vi "Get Recording.vi"(8 "error in":errorcluster, 9 "Get":bool, 10 "Recording":fxp<+/-,8,8>[](array[numeric]), 11 "Interface In":T1) -> (0 "error out":errorcluster, 1 "Get?":bool, 3 "Interface Out":T1)   [LabVIEW 2015]
uses:
  TypeDefs Host/FPGA Dynamic Interface.ctl
  TypeDefs Host/Open Audio FGV Enum.ctl
  <vilib>/Utility/error.llb/Error Cluster From Error Code.vi
  <vilib>/rvi/errors/niLvFpgaAdjustHostInterfaceError.vi
  <vilib>/rvi/interface/common/niFpgaWaitOnOcc.vi
  <vilib>/rvi/interface/nirviReadWriteControl/nirviReadWriteControl.xnode
  <vilib>/rvi/interface/nirviMethod/nirviMethod.xnode
  <vilib>/rvi/errors/niLvFpgaMergeErrorWithErrorCode.vi
  <vilib>/FPGAPlugInAG/Dynamic/niLvFpga_WriteFifo_Dynamic.vi
  NiFpgaLv.dll
  <vilib>/rvi/interface/Simulation/niFpgaSimulationCallBeginRW.vi
  <vilib>/FPGAPlugInAG/Dynamic/niLvFpga_ConfigureFifo_Dynamic.vi
  <vilib>/FPGAPlugInAG/Dynamic/niLvFpga_StartFifo_Dynamic.vi
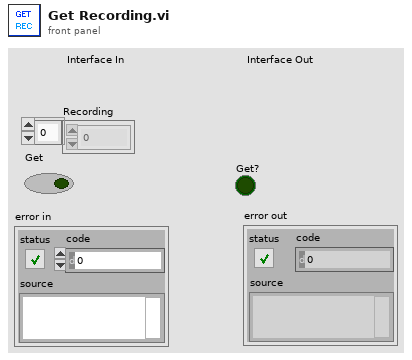
[diagram p1: front panel]
types:
  T1 = typedef "FPGA Dynamic Interface.ctl" = refnum<k20>
  T2 = typedef "Open Audio FGV Enum.ctl" = enum16{"Get", "Set"}
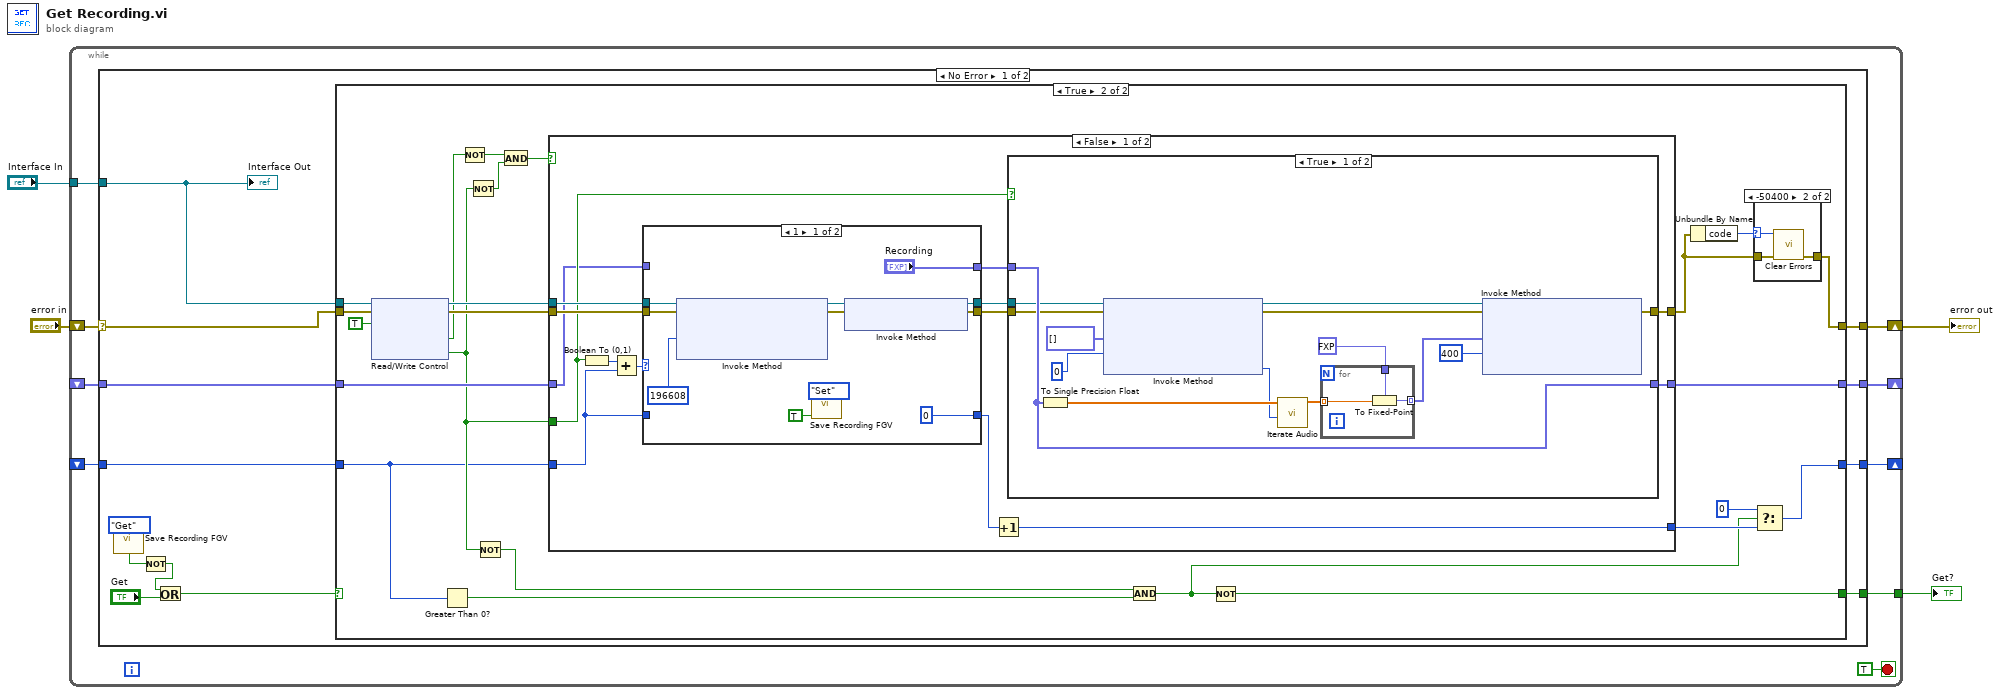
[diagram p0: block diagram]
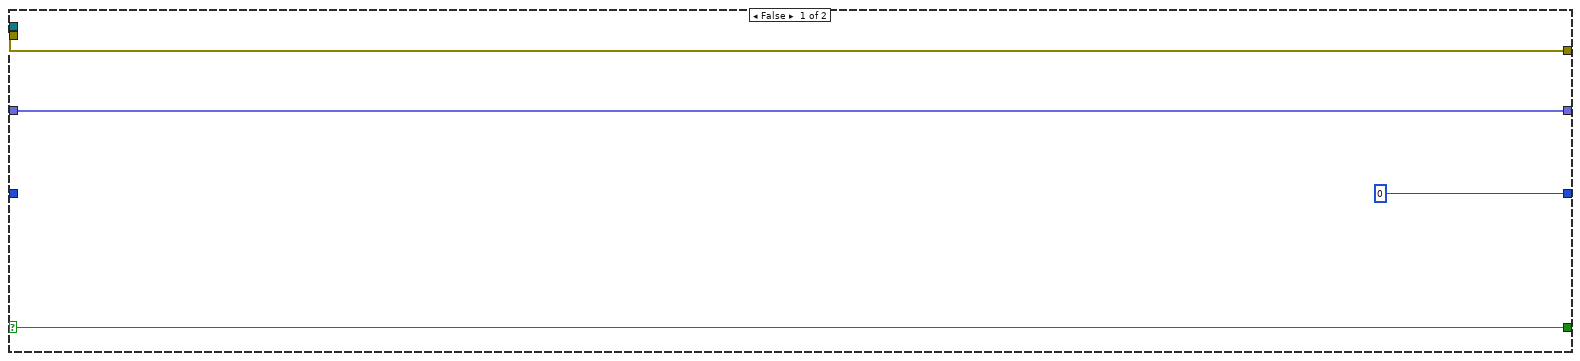
[diagram p2: hidden frame]
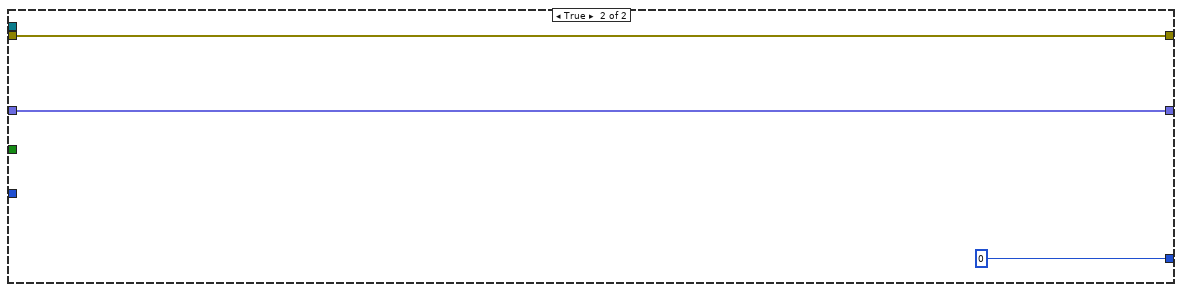
[diagram p6: hidden frame]
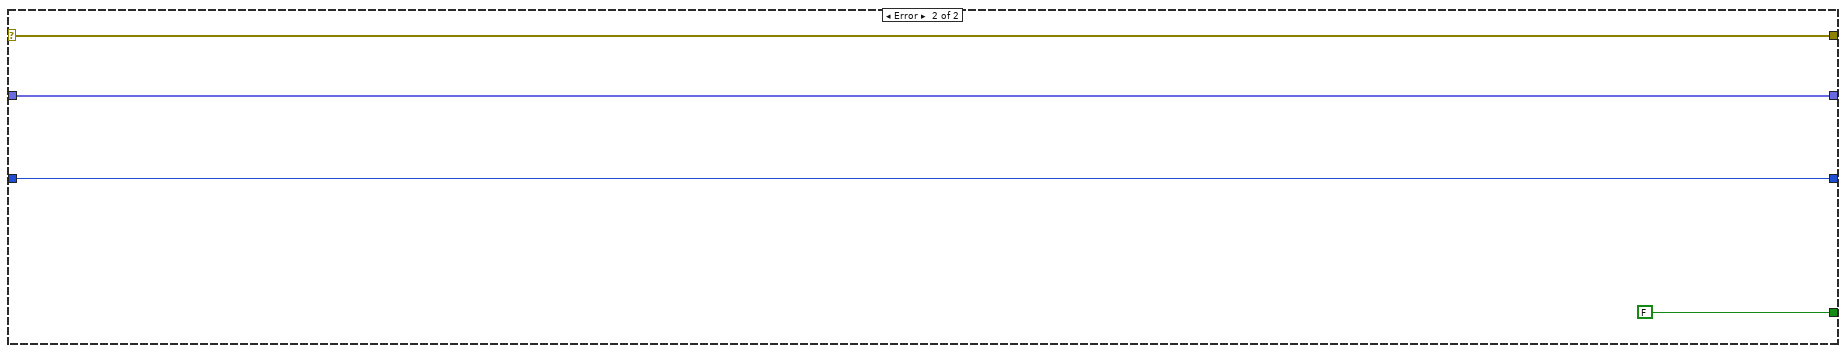
[diagram p7: hidden frame]
diagram:
  n1 = while {
    shift-right: [w9] -> w3
    shift-left: "error in" -> [w6]
    shift-right: [w13] -> _
    shift-left: _ -> [w11]
    shift-right: [w10] -> _
    shift-left: _ -> [w12]
    tunnel: [w7] -> w4
    tunnel: "Interface In" -> [w5]
    stop <- TRUE stop-if-true
    n2 = case shown="No Error" w6 {
      selector: w6 -> [w15 w112]
      tunnel: [w26 w111] -> w13
      tunnel: w12 -> [w25 w110]
      tunnel: w11 -> [w24 w111]
      tunnel: [w23 w110] -> w10
      tunnel: [w22 w112] -> w9
      tunnel: [w21 FALSE] -> w7
      tunnel: w5 -> [w14 _]
      frame No Error {
        n3 = call "Save Recording FGV.vi"("Command"=Open_Audio_FGV_Enum."Get") -> ("Save?"=w17:bool)  [unwired: 10 in]
        n4 = Not(x=w17) -> (.not. x?=w16:bool)
        n5 = Or(x=w16, y="Get") -> (x .or. y?=w19:bool)
        n6 = case shown="True" w19 {
          selector: w19 -> [w28 _]
          tunnel: [w29 w53] -> w26
          tunnel: w15 -> [w30 w51]
          tunnel: w25 -> [_ w33]
          tunnel: w24 -> [w29 w47]
          tunnel: [0 ("Chunk size") w41] -> w23
          tunnel: [w30 w42] -> w22
          tunnel: [w28 w38] -> w21
          tunnel: w14 -> [_ w31]
          frame False {
          }
          frame True {
            n7 = xnode "Read/Write Control"("FPGA VI Reference In"=w31, "error in"=w51, "Init?"=TRUE) -> ("FPGA VI Reference Out"=w52:T1, "error out"=w50:errorcluster, "To Host?"=w36:bool, "From Host?"=w35:bool)
            n8 = Greater Than 0?(x=w33) -> (x > 0?=w32:bool)
            n9 = Not(x=w36) -> (.not. x?=w49:bool)
            n10 = Not(x=w35) -> (.not. x?=w48:bool)
            n11 = Not(x=w35) -> (.not. x?=w34:bool)
            n12 = And(x=w49, y=w48) -> (x .and. y?=w45:bool)
            n13 = case shown="False" w45 {
              tunnel: w50 -> [w71 w107]
              tunnel: [w60 w107] -> w43
              tunnel: [w65 w108] -> w53
              tunnel: w47 -> [w61 w108]
              tunnel: w52 -> [w70 _]
              tunnel: w35 -> [w64 _]
              tunnel: w33 -> [w59 _]
              tunnel: [w62 0 ("Chunk size")] -> w46
              frame False {
                n14 = Boolean To (0,1)(Boolean=w64) -> (0, 1=w67:i16)
                n15 = Add(x=w67, y=w59) -> (x+y=w66:i32)
                n16 = case shown="1" w66 {
                  tunnel: w71 -> [w101 w104]
                  tunnel: w70 -> [w100 w105]
                  tunnel: [w97 w105] -> w69
                  tunnel: [w96 w104] -> w68
                  tunnel: w61 -> [_ w103]
                  tunnel: ["Recording" w103] -> w63
                  tunnel: w59 -> [_ w102]
                  tunnel: [0 ("Chunk size") w102] -> w58
                  frame 1 {
                    n17 = xnode "Invoke Method"("FPGA VI Reference In"=w100, "error in"=w101, "Requested Depth"=u32 196608) -> ("FPGA VI Reference Out"=w98:T1, "error out"=w95:errorcluster)  [unwired: 1 out]
                    n18 = call "Save Recording FGV.vi"("Command"=Open_Audio_FGV_Enum."Set", "Save"=TRUE) -> ()  [unwired: 9 in, 1 out]
                    n19 = xnode "Invoke Method"("FPGA VI Reference In"=w98, "error in"=w95) -> ("FPGA VI Reference Out"=w97:T1, "error out"=w96:errorcluster)
                  }
                  frame 0, Default {
                  }
                }
                n20 = Increment(x=w58) -> (x+1=w62:i32)
                n21 = case shown="True" w64 {
                  tunnel: [w85 w89] -> w60
                  tunnel: w69 -> [w78 _]
                  tunnel: w68 -> [w77 w89]
                  tunnel: [w83 w90] -> w65
                  tunnel: w63 -> [w83 w90]
                  frame True {
                    n22 = To Single Precision Float(number=w83) -> (single precision float=w84:sgl[])
                    n23 = xnode "Invoke Method"("FPGA VI Reference In"=w78, "error in"=w77, "Data"=fxp<+/-,8,8>[] [], "Timeout (ms)"=0) -> ("FPGA VI Reference Out"=w76:T1, "error out"=w75:errorcluster, "Empty Elements Remaining"=w72:u32)
                    n24 = call "Iterate Audio.vi"("Chunk size"=w72, "Msg"=w84) -> ("Subarray"=w82:sgl[])  [unwired: 8 in, 1 out]
                    n25 = for {
                      tunnel: [w88] -> w79 mode=indexing
                      tunnel: w82 -> [w87] mode=indexing
                      tunnel: fxp<+/-,8,8> 0.0 ("Numeric") -> [w86]
                      n26 = To Fixed-Point(fixed-point type=w86, number=w87) -> (fixed-point=w88:fxp<+/-,8,8>)
                    }
                    n27 = xnode "Invoke Method"("FPGA VI Reference In"=w76, "error in"=w75, "Data"=w79, "Timeout (ms)"=400) -> ("error out"=w85:errorcluster)  [unwired: 2 out]
                  }
                  frame False {
                  }
                }
              }
              frame True {
              }
            }
            n28 = And(x=w34, y=w32) -> (x .and. y?=w39:bool)
            n29 = Not(x=w39) -> (.not. x?=w38:bool)
            n30 = Unbundle By Name(w43) -> ("code"=w44:i32)
            n31 = case shown="-50400" w44 {
              selector: w44 -> [_ w57]
              tunnel: w43 -> [w54 w56]
              tunnel: [w54 w55] -> w42
              frame 0, Default {
              }
              frame -50400 {
                n32 = call <vilib>:"Clear Errors.vi"("error in (no error)"=w56, "specific error code to clear (0: all)"=w57) -> ("error out"=w55:errorcluster)  [unwired: 4 in, 1 out]
              }
            }
            n33 = Select(t=0, s=w39, f=w46) -> (s? t:f=w41:i32)
          }
        }
        "Interface Out" <- w14
      }
      frame Error {
      }
    }
  }
  "error out" <- w3
  "Get?" <- w4
